vi "Test Find Two Common Chars.vi"(11 "Test Case In":refnum<class "Common Section Finder Test.lvclass">) -> (0 "error out":errorcluster, 3 "Test Case Out":refnum<class "Common Section Finder Test.lvclass">)   [LabVIEW 2020, in "Common Section Finder Test.lvclass"]
uses:
  Common Section Finder Test.lvclass
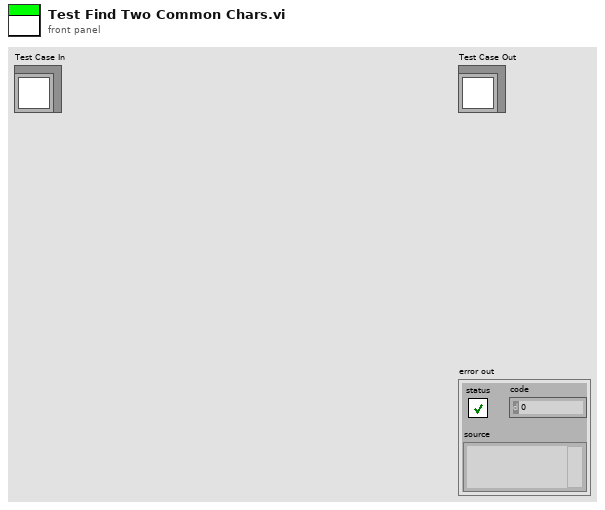
[diagram p1: front panel]
types:
  T1 = cluster{"Selection Start":u32, "Selection End":u32}
  T2 = cluster{"Selection Start":u32, "Selection End":u32}[]
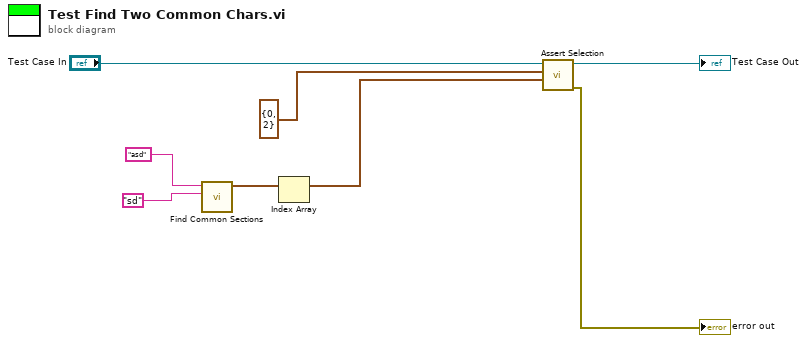
[diagram p0: block diagram]
diagram:
  n1 = call "Find Common Sections.vi"("Reference"="sd", "Target"="asd") -> ("Sections in Reference"=w3:T2)  [unwired: 9 in]
  n2 = Index Array(array=w3) -> (element=w2:T1)  [unwired: 1 in]
  n3 = call "Assert Selection.vi"("Actual"=w2, "Expected"=T1 {"Selection Start"=0, "Selection End"=2}, "Added Section Finder Test In"="Test Case In") -> ("error out"=→"error out":errorcluster, "Added Section Finder Test Out"=→"Test Case Out":refnum<class "Common Section Finder Test.lvclass">)  [unwired: 7 in]
